vi "Write ListItems.vi"(8 "error in (no error)":errorcluster, 10 "List Items":string[](array[string]), 11 "ScrollingList in":refnum<class "ScrollingList.lvclass">) -> (0 "error out":errorcluster, 3 "ScrollingList out":refnum<class "ScrollingList.lvclass">)   [LabVIEW 2020, in "ScrollingList.lvclass"]
uses:
  ScrollingList.lvclass
  ScrollingList.lvclass/ScrollingList.ctl
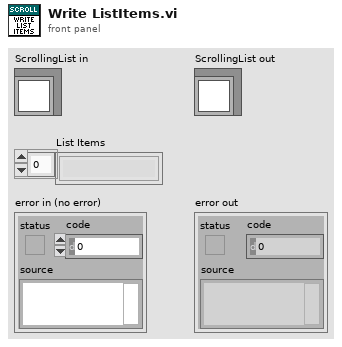
[diagram p1: front panel]
types:
  T1 = typedef "ScrollingList.lvclass/State Data.ctl" = cluster{"Timeout":i32, "Time":timestamp, "Y":i32, "Origin:Top":i16, "Rate":dbl, "ListItems":string[], "Item Height":i32, "Max Height":i32}
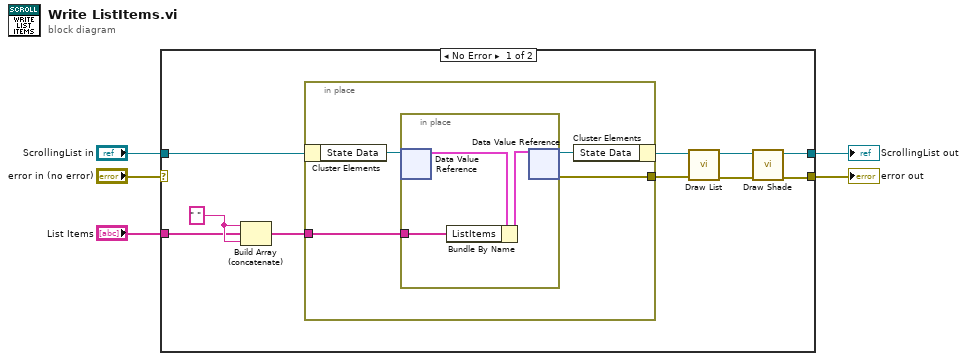
[diagram p0: block diagram]
diagram:
  n1 = case shown="No Error" "error in (no error)" {
    selector: "error in (no error)" -> [_ w24]
    tunnel: [w6 w24] -> w4
    tunnel: [w8 w23] -> w2
    tunnel: "ScrollingList in" -> [w13 w23]
    tunnel: "List Items" -> [w14 _]
    frame No Error {
      w15 = " "
      n2 = Build Array (concatenate)(w15, w14, w15) -> (w12:string[])
      n3 = in-place {
        in-place-border: w12 -> [w18]
        in-place-border: [w16] -> w10
        n4 = in-place-cluster #1(w13) -> ("State Data"=w19:refnum<data-value>)
        n5 = in-place {
          in-place-border: w18 -> [w21]
          n6 = in-place-dvr #2(w19) -> (w22:T1)  [unwired: 1 out]
          n7 = Bundle By Name(cluster=w22, "ListItems"=w21) -> (w20:T1)
          n8 = in-place-dvr #2(w20) -> (w17:refnum<data-value>, w16:errorcluster)
        }
        n9 = in-place-cluster #1("State Data"=w17) -> (w11:refnum<class "ScrollingList.lvclass">)
      }
      n10 = call "Draw List.vi"("error in (no error)"=w10, "ScrollingList in"=w11) -> ("error out"=w7:errorcluster, "ScrollingList out"=w9:refnum<class "ScrollingList.lvclass">)  [unwired: 8 in]
      n11 = call "Draw Shade.vi"("error in (no error)"=w7, "ScrollingList in"=w9) -> ("error out"=w6:errorcluster, "ScrollingList out"=w8:refnum<class "ScrollingList.lvclass">)  [unwired: 8 in]
    }
    frame Error {
    }
  }
  "error out" <- w4
  "ScrollingList out" <- w2
